vi "PCO_GetSoftFPS.vi"(0 "ph":u64, 5 "error in (no error)":errorcluster {"code" format="%x"}) -> (14 "ph_out":u64, 15 "ErrorMessage":i32 format="%x", 16 "dwFPS":u32, 17 "dwExp":u32, 18 "wTimeBaseExp":u16(ring) items=["ns", "us", "ms"], 19 "error out":errorcluster {"code" format="%x"})   [LabVIEW 2019, in "SDK.lvlib" / "TimingControl.lvlib"]
doc: "Gets the timing for the specified FPS (frames per second). The FPS is set by running an iterative loop, so reponse time may be slow."
uses:
  TimingControl.lvlib
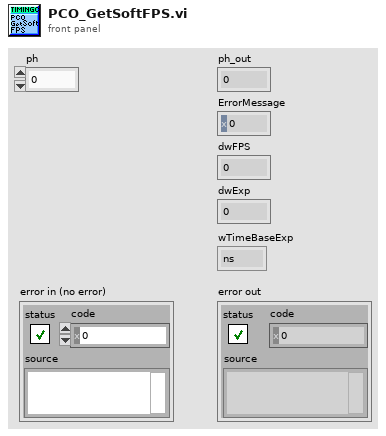
[diagram p1: front panel]
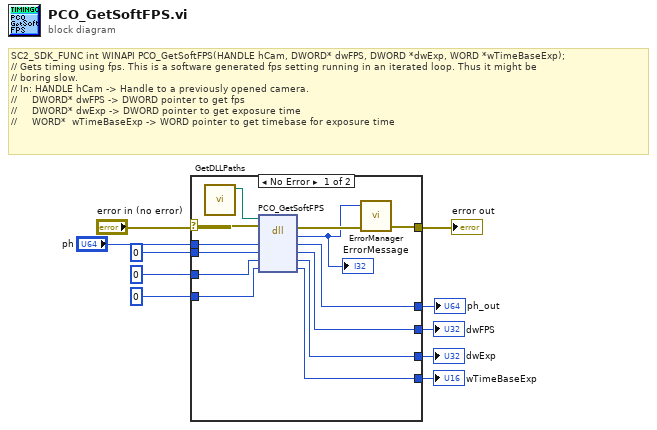
[diagram p0: block diagram]
diagram:
  # "SC2_SDK_FUNC int WINAPI PCO_GetSoftFPS(HANDLE hCam, DWORD* dwFPS, DWORD *dwExp, WORD *wTimeBaseExp);\n// Gets timing using fps. This is a software generated fps setting running in an iterated loop. Thus it might be\n// boring slow.\n// In: HANDLE hCam -> Handle to a previously opened camera.\n//     DWORD* dwFPS -> DWORD pointer to get fps\n//     DWORD* dwExp -> DWORD pointer to get exposure time\n//     WORD*  wTimeBaseExp -> WORD pointer to get timebase for exposure time"
  n1 = case shown="No Error" "error in (no error)" {
    selector: "error in (no error)" -> [w19 w28]
    tunnel: "ph" -> [w23 w27]
    tunnel: u32 0 ("wFrameRateStatus") -> [w22 w26]
    tunnel: u32 0 ("dwFrameRate") -> [w21 w25]
    tunnel: u16 0 ("dwFrameRateExposure") -> [w20 w24]
    tunnel: [w17 w28] -> w6
    tunnel: [w14 w27] -> w4
    tunnel: [w13 w26] -> w3
    tunnel: [w12 w25] -> w2
    tunnel: [w11 w24] -> w1
    frame No Error {
      n2 = call "GetDLLPaths.vi"() -> ("SC2_Cam_Path"=w15:path)  [unwired: 8 in, 3 out]
      n3 = dll-call lib="?" fn="PCO_GetSoftFPS"(path in=w15, error in=w19, "ph"=w23, "dwFPS"=w22, "dwExp"=w21, "wTimeBaseExp"=w20) -> (error out=w18:errorcluster, "return type"=w16:i32, "ph"=w14:u64, "dwFPS"=w13:u32, "dwExp"=w12:u32, "wTimeBaseExp"=w11:u16)  [unwired: 1 in, 1 out]
      "ErrorMessage" <- w16
      n4 = call "ErrorManager.vi"("error in (no error)"=w18, "error code"=w16) -> ("error out"=w17:errorcluster)  [unwired: 2 in, 1 out]
    }
    frame Error {
    }
  }
  "error out" <- w6
  "ph_out" <- w4
  "dwFPS" <- w3
  "dwExp" <- w2
  "wTimeBaseExp" <- w1
